vi "Example_OE2031&OE2041 Trig in_double_char.vi"() -> ()   [LabVIEW 2011]
panel:
  out "Wave":cluster{"Parameter":dbl, "Parameter":dbl}(graph)
  in  "Parameter Index2":u16(ring)=1 items=["X", "Y", "R", "θ", "Frequency", "XD1", "YD1", "RD1", "θD1", "XD2", "YD2", "RD2", "θD2", "XD3", "YD3", "RD3", "θD3", "X_Noise", "Y_Noise", "AUXADC1", "AUXADC2", "AUXADC3", "AUXADC4"]
  out "data_buffer":dbl[][](array[numeric])
  out "loss count":i32=-1
  out "cnt":u16
  in  "Ref_Source":u8(ring)=1 items=["External", "Internal"]
  in  "Interval Count":u32=1 min=1 max=100000
  in  "选项卡控件":enum32{"选项卡 "}(tab)
  in  "Sweep Mode":u16(ring) items=["Linear", "Log"]
  in  "Start Frequency(Hz)":dbl=1000.0 min=1e-05 max=60000000.0 format="%#.3f"
  in  "Stop Frequency(Hz)":dbl=5000.0 min=1e-05 max=60000000.0 format="%#.3f"
  in  "Linear Step Frequency(Hz)":dbl=1000.0 min=1e-05 max=60000000.0 format="%#.3f"
  in  "Log Step Percent(%)":dbl=10.0 min=-100.0 max=100.0 format="%#.2f"
  in  "Step Time(ms)":i32=1000 min=50 max=100000
  in  "Sweep Run Mode":u16(ring) items=["Stop", "Singal", "Loop"]
  out "Group":u32
  in  "Sweep":u16(ring) items=["OFF", "ON"]
  in  "function":T1(ring)
  in  "Parameter Index":u16(ring) items=["X", "Y", "R", "θ", "Frequency", "XD1", "YD1", "RD1", "θD1", "XD2", "YD2", "RD2", "θD2", "XD3", "YD3", "RD3", "θD3", "X_Noise", "Y_Noise", "AUXADC1", "AUXADC2", "AUXADC3", "AUXADC4"]
  in  "IP Address":string="192.168.1.10"
  in  "Timeout":u32=100
  in  "Port":u32=10001
  in  "Connect":bool
  in  "Trig Mode":u8(ring) items=["Internal", "Ext_Rissing_Edge", "Ext_Falling_Edge", "Ext_High_Level", "Ext_Low_Level"]
  out "Error out":errorcluster caption="error out"
  in  "Remote Mode":u16(ring) items=["USB"=0, "Ethernet"=3]
  in  "VISA resource name":refnum<visa-resource-name>
  # "Tel          :   +86-020-84133345\nWebsite  :   www.ssi-instrument.com\nE-mail     :   support@si-instrument.com"
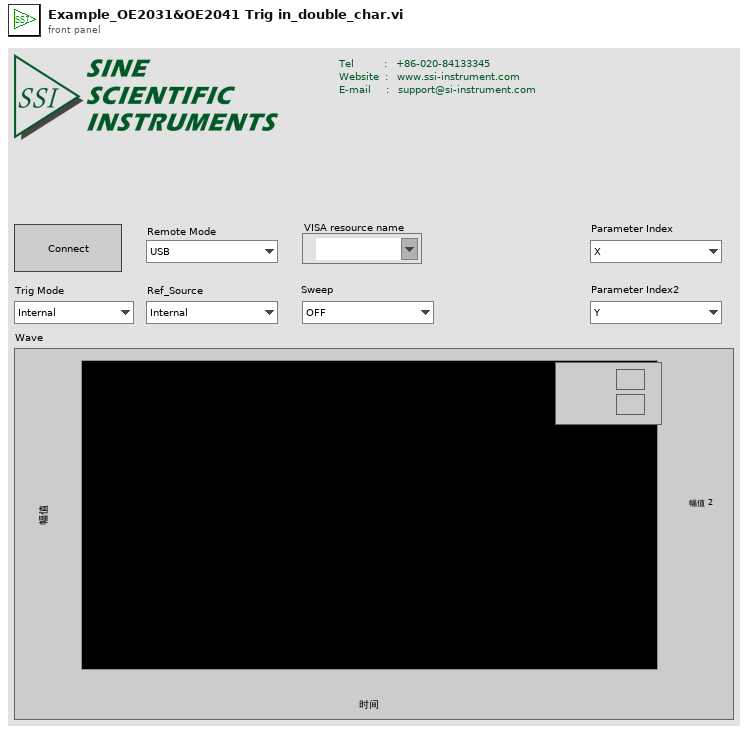
[diagram p1: front panel]
types:
  T1 = enum16{"initial", "Trig In Type", "Sample", "Ext_Sweep_Trig In", "Int_Sweep_Trig In"}
  T2 = enum8{"Enabled", "Disabled", "Disabled and Grayed Out"}
  T3 = cluster{"Port":u32, "Timeout":u32, "IP Address":string}
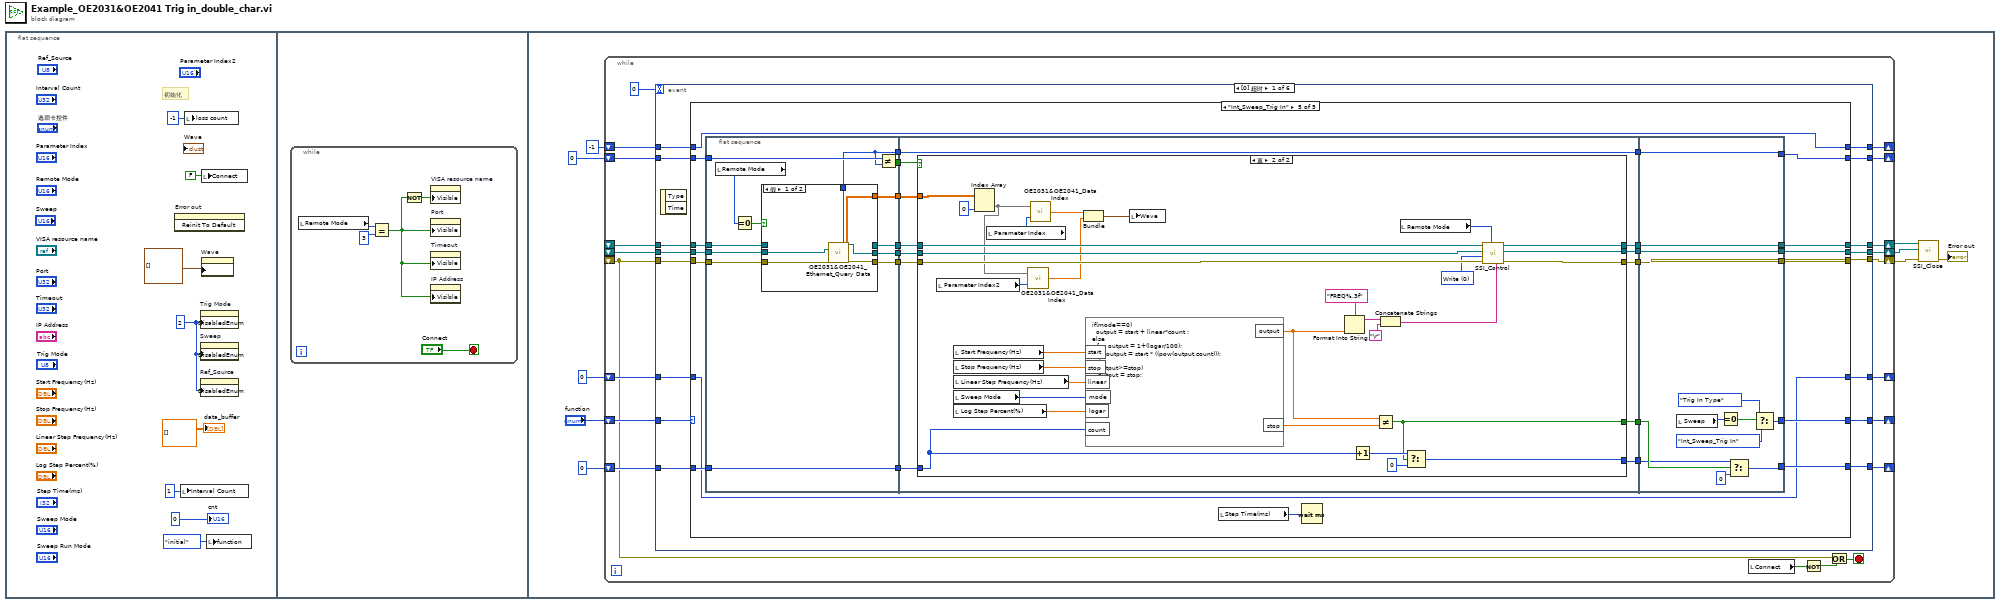
[diagram p0: block diagram]
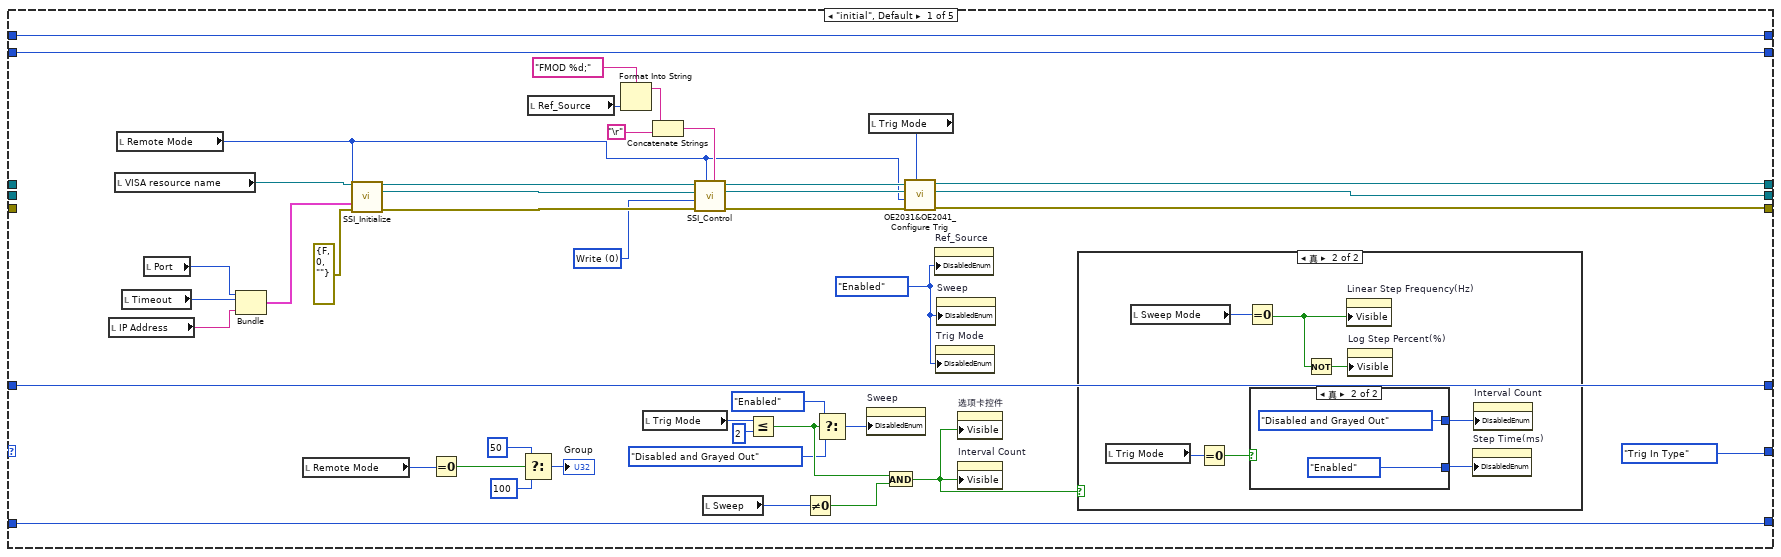
[diagram p2: hidden frame]
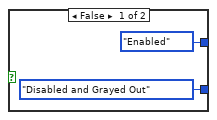
[diagram p4: hidden frame]
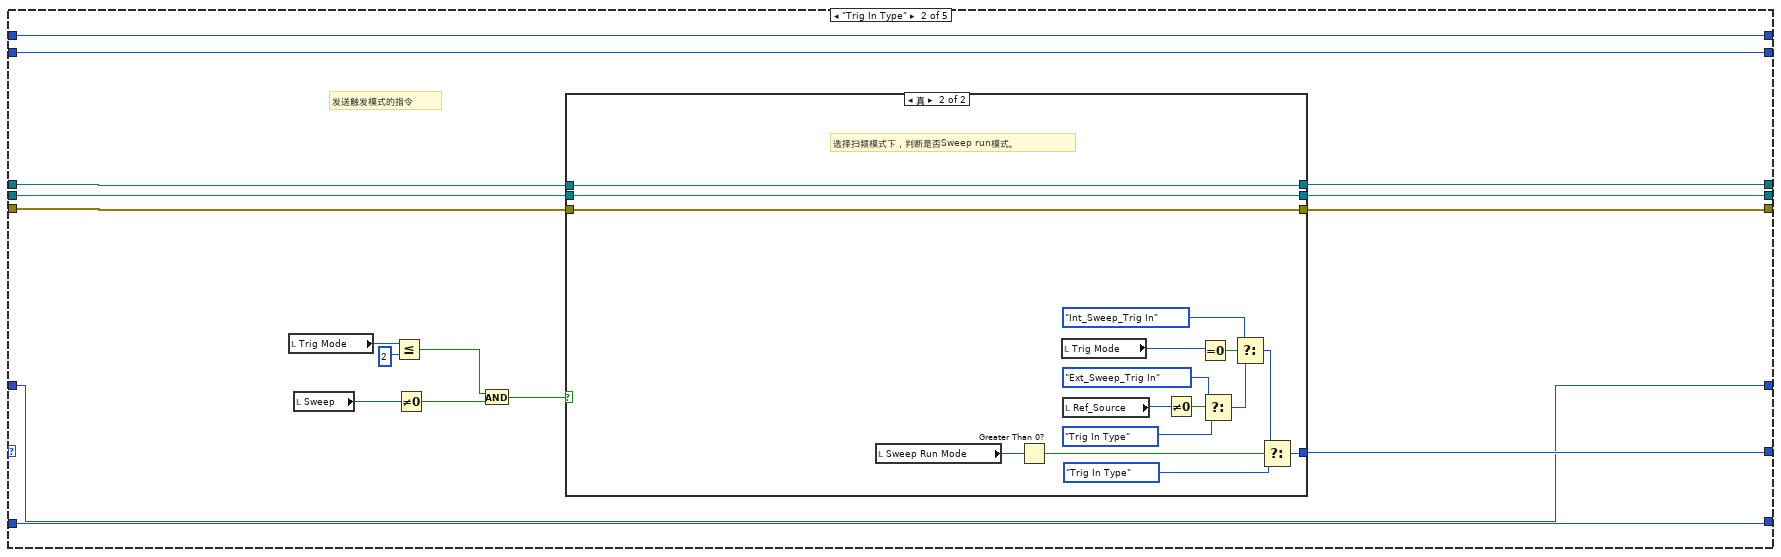
[diagram p5: hidden frame]
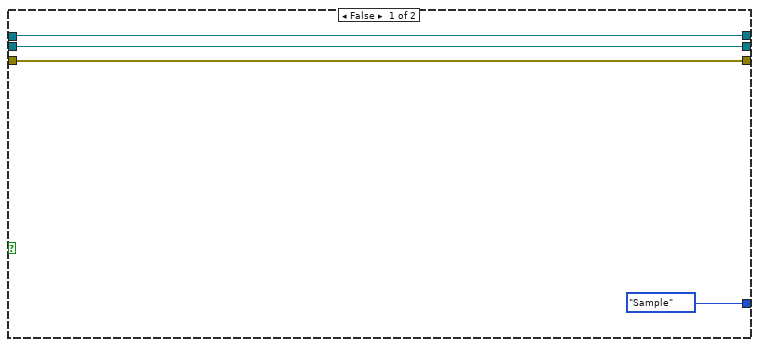
[diagram p6: hidden frame]
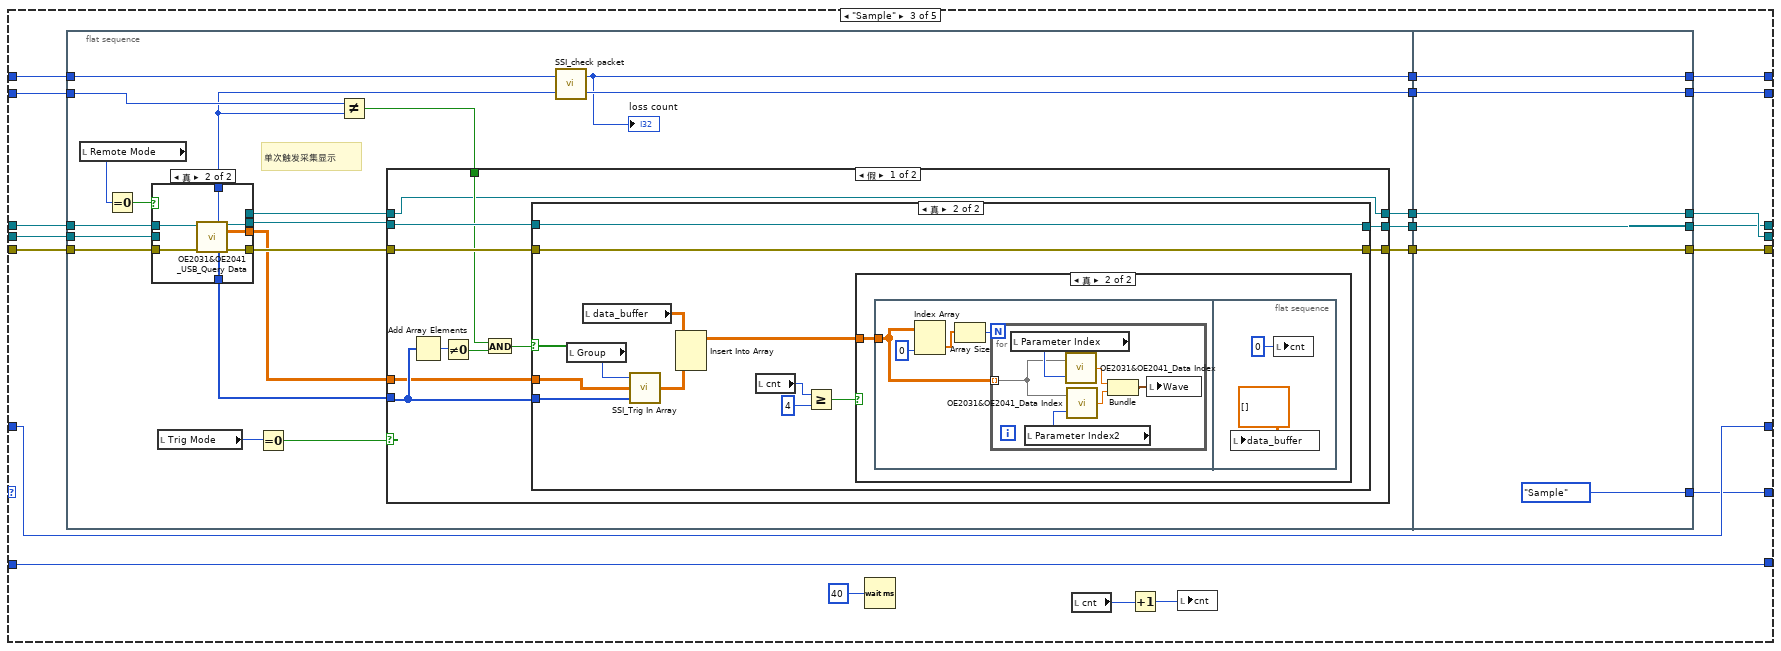
[diagram p7: hidden frame]
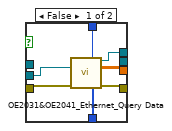
[diagram p8: hidden frame]
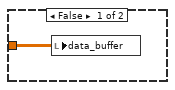
[diagram p10: hidden frame]
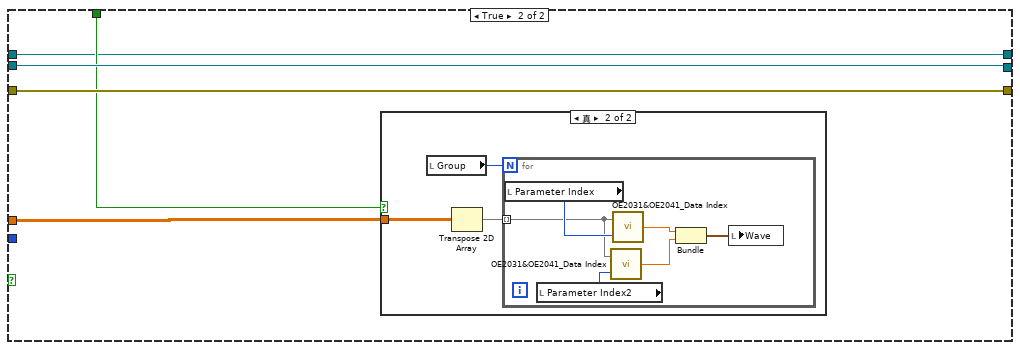
[diagram p11: hidden frame]
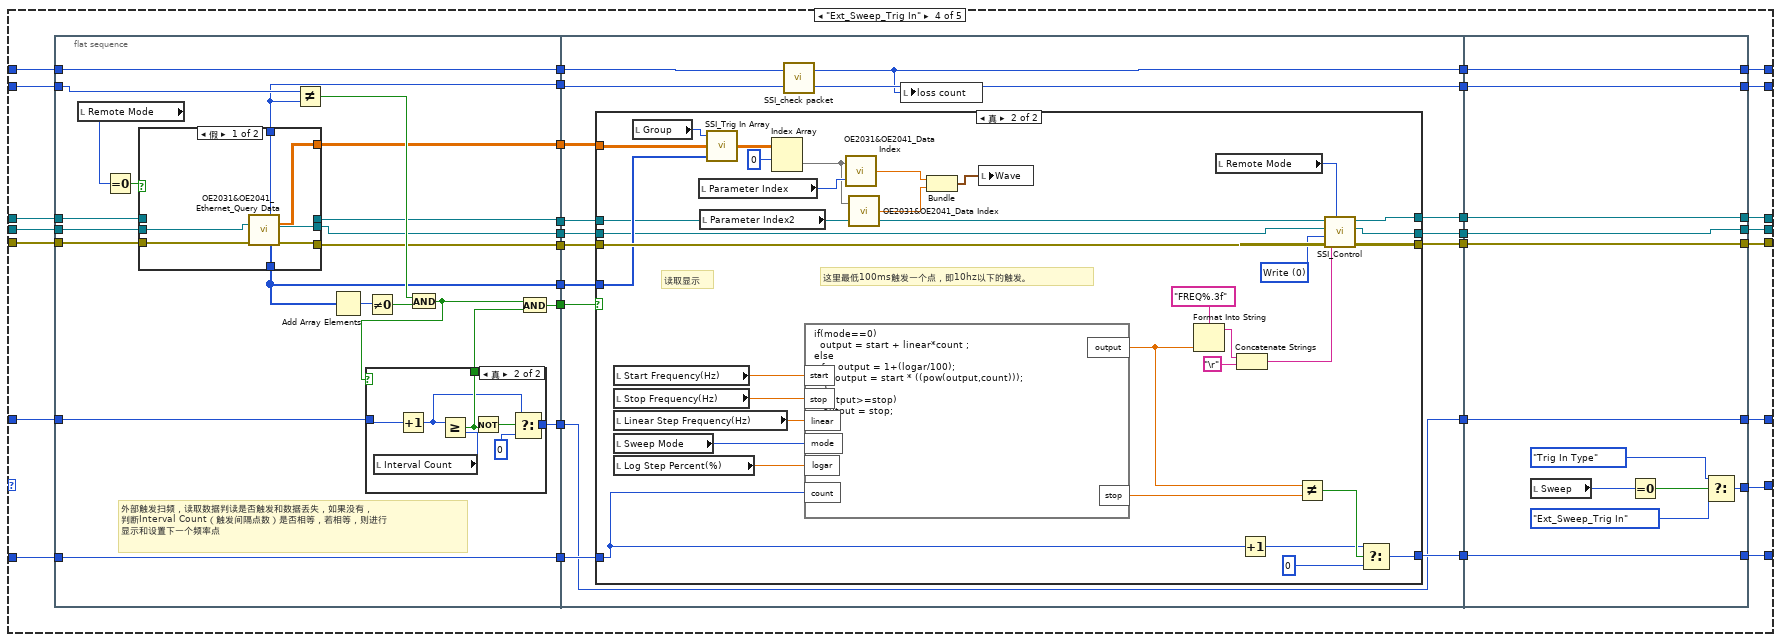
[diagram p13: hidden frame]
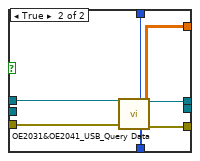
[diagram p14: hidden frame]
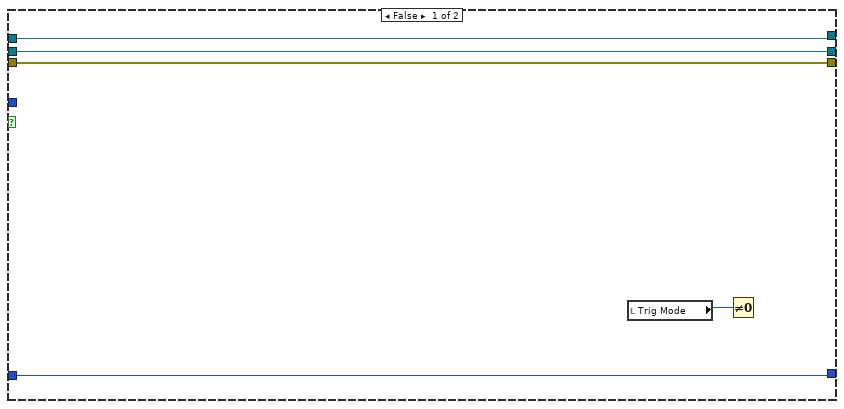
[diagram p16: hidden frame]
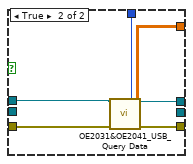
[diagram p17: hidden frame]
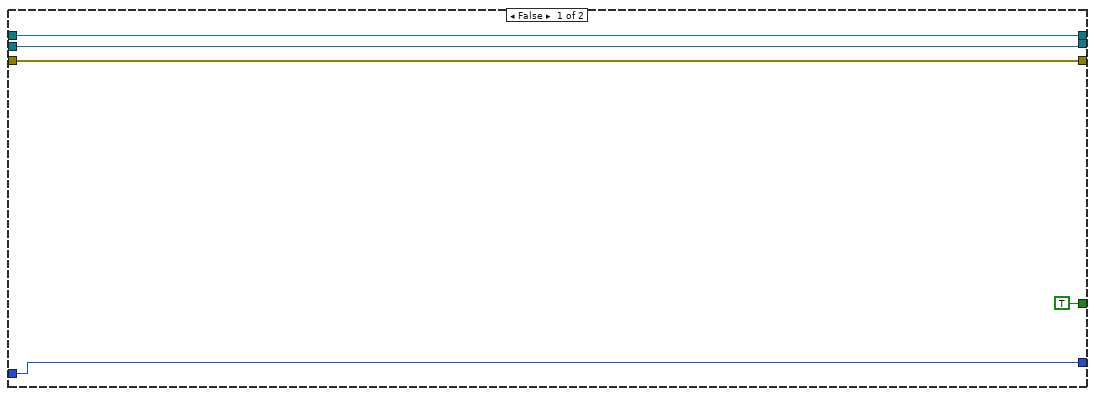
[diagram p18: hidden frame]
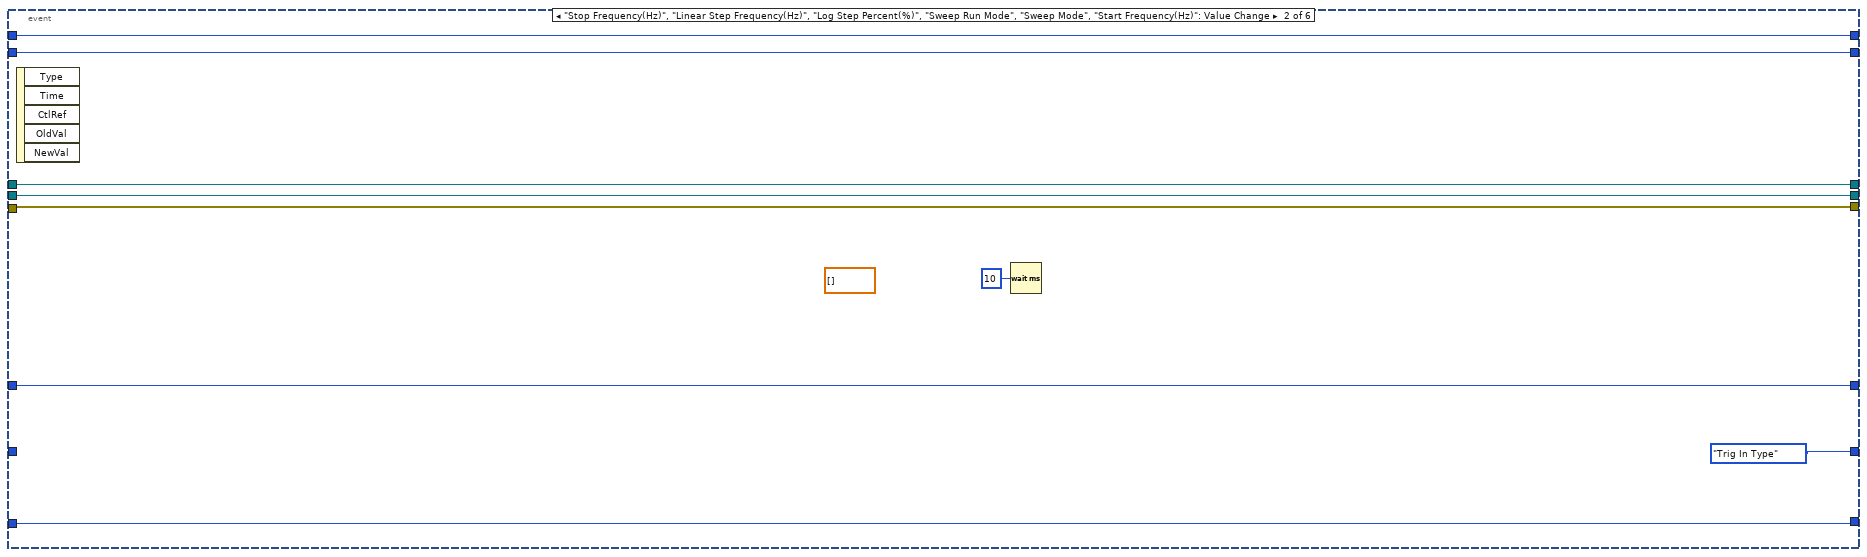
[diagram p19: hidden frame]
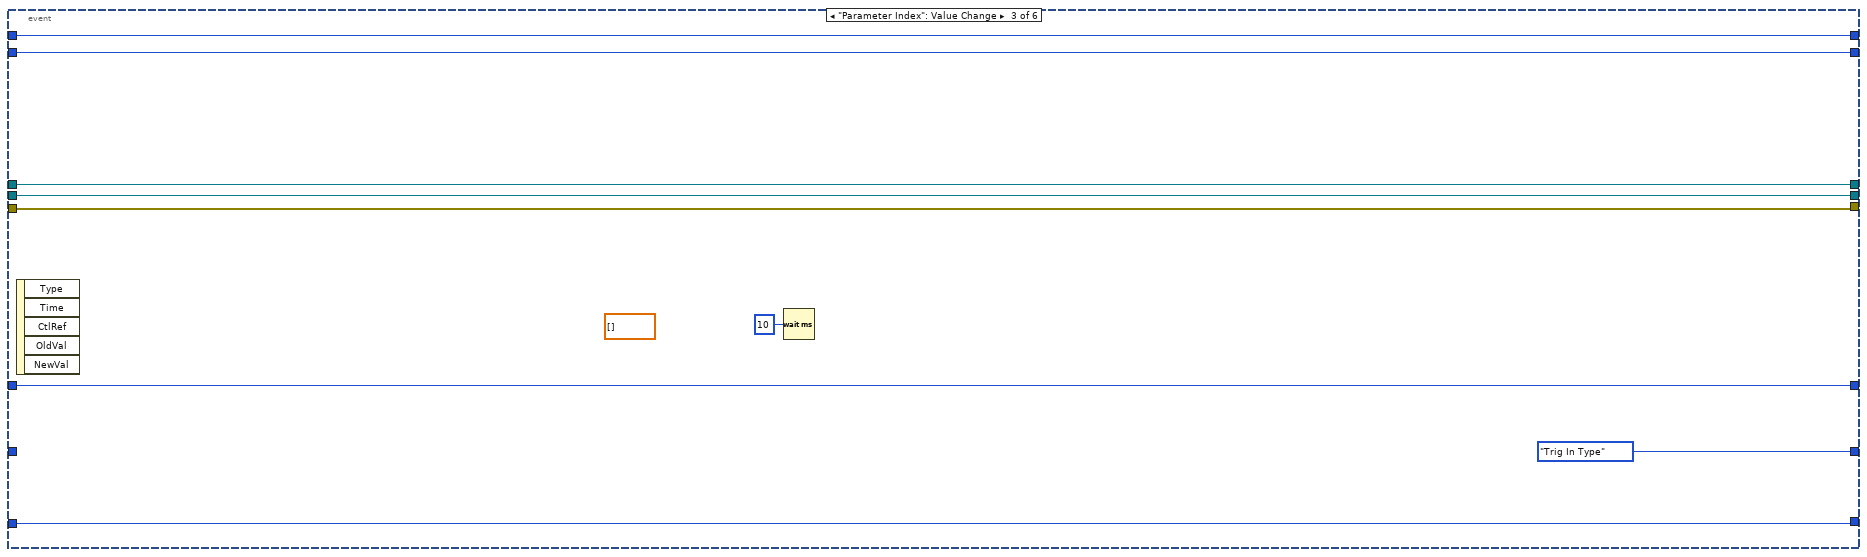
[diagram p20: hidden frame]
diagram:
  n1 = flat-sequence {
    frame #0 {
      w3 = 2
      # "初始化"
      n2 = invoke on="Error out" class="Clust (严格)" method="Reinit To Default"() -> ()  [unwired: 3 in, 3 out]
      n3 = local write "Interval Count"(u32 1 ("Interval Count")) -> ()
      n4 = local write "loss count"(-1 ("loss count")) -> ()
      n5 = property on="Trig Mode" class="Ring (严格)"("DisabledEnum"=w3) -> ()  [unwired: 2 in, 2 out]
      n6 = property on="Sweep" class="Ring (严格)"("DisabledEnum"=w3) -> ()  [unwired: 2 in, 2 out]
      n7 = property on="Ref_Source" class="Ring (严格)"("DisabledEnum"=w3) -> ()  [unwired: 2 in, 2 out]
      n8 = local write "Connect"(FALSE ("Connect")) -> ()
      n9 = property on="Wave" class="WFChart (严格)"("History Data"=cluster{"Parameter":dbl, "Parameter":dbl}[] [] ("历史数据")) -> ()  [unwired: 2 in, 2 out]
      n10 = local write "function"(T1."initial" ("function")) -> ()
      "data_buffer" <- dbl[][] []
      "cnt" <- 0
    }
    frame #1 {
      n11 = while {
        stop <- "Connect" stop-if-true
        n12 = local read "Remote Mode"() -> (w12:u16)
        n13 = Equal?(x=w12, y=u16 3) -> (x = y?=w10:bool)
        n14 = Not(x=w10) -> (.not. x?=w9:bool)
        n15 = property on="VISA resource name" class="VISAName"("Visible"=w9) -> ()  [unwired: 2 in, 2 out]
        n16 = property on="Port" class="DigNum (严格)"("Visible"=w10) -> ()  [unwired: 2 in, 2 out]
        n17 = property on="Timeout" class="DigNum (严格)"("Visible"=w10) -> ()  [unwired: 2 in, 2 out]
        n18 = property on="IP Address" class="Str"("Visible"=w10) -> ()  [unwired: 2 in, 2 out]
      }
    }
    frame #2 {
      n19 = while {
        shift-right: [w37] -> _
        shift-left: "function" -> [w38]
        shift-right: [w35] -> _
        shift-left: 0 ("f") -> [w36]
        shift-right: [w32] -> _
        shift-left: 0 -> [w33]
        shift-right: [w29] -> _
        shift-left: 0 -> [w30]
        shift-right: [w26] -> w16
        shift-left: _ -> [w40]
        shift-right: [w39] -> w21
        shift-left: _ -> [w28]
        shift-right: [w27] -> w17
        shift-left: _ -> [w25]
        shift-right: [w23] -> _
        shift-left: -1 ("loss count") -> [w24]
        stop <- w41 stop-if-true
        n20 = event shown="[0] 超时" {
          selector: _ -> [_ _ _ _ _ _]
          dyn-events: _ -> [_ _ _ _ _ _]
          timeout: 0 -> [_ _ _ _ _ _]
          tunnel: w40 -> [w58 w524 w536 w554 w578 w597]
          tunnel: [w57 w524 w536 w549 w577 w597] -> w26
          tunnel: [w56 w522 w535 w551 w580 w598] -> w39
          tunnel: w28 -> [w55 w522 w535 w556 w581 w598]
          tunnel: w38 -> [w54 _ _ _ w584 _]
          tunnel: [w53 T1."Trig In Type" ("function") T1."Trig In Type" ("function") T1."Trig In Type" ("function") w584 T1."Trig In Type" ("function")] -> w37
          tunnel: w36 -> [w52 w528 w537 w560 w585 w593]
          tunnel: [w51 w528 w537 w560 w585 w593] -> w35
          tunnel: w33 -> [w50 w526 w533 w558 w582 w595]
          tunnel: [w49 w526 w533 w558 w582 w595] -> w32
          tunnel: w30 -> [w48 w520 w532 w559 w583 w592]
          tunnel: [w47 w520 w532 w559 w583 w592] -> w29
          tunnel: [w46 w523 w530 w550 w576 w596] -> w27
          tunnel: w25 -> [w45 w523 w530 w555 w579 w596]
          tunnel: w24 -> [w44 w525 w529 w538 w572 w594]
          tunnel: [w43 w525 w529 w538 w572 w594] -> w23
          event Timeout {
            n21 = event-data() -> ()  [unwired: 1 in, 2 out]
            n22 = case shown="\"Int_Sweep_Trig In\"" w54 {
              tunnel: w58 -> [_ w129 w169 w294 w417]
              tunnel: w55 -> [_ w127 w168 w293 w416]
              tunnel: [w80 w128 w152 w290 w430] -> w57
              tunnel: [w78 w126 w160 w291 w429] -> w56
              tunnel: [T1."Trig In Type" ("function") w125 w166 w279 w427] -> w53
              tunnel: w52 -> [w95 w124 w170 w292 w428]
              tunnel: [w95 w124 w170 w289 w426] -> w51
              tunnel: w50 -> [w93 w123 w165 w288 w432]
              tunnel: [w93 w123 w163 w287 w431] -> w49
              tunnel: w48 -> [w94 w122 w167 w274 w425]
              tunnel: [w94 w122 w167 w271 w425] -> w47
              tunnel: [w79 w114 w153 w267 w408] -> w46
              tunnel: w45 -> [_ w115 w155 w270 w412]
              tunnel: w44 -> [w60 w113 w158 w266 w407]
              tunnel: [w60 w113 w151 w263 w407] -> w43
              frame "initial", Default {
                w59 = T2."Enabled" ("禁用")
                w72 = u16 0 items=["Write", "Read"] ("Control")
                n23 = local read "IP Address"() -> (w75:string)
                n24 = local read "VISA resource name"() -> (w81:refnum<visa-resource-name>)
                n25 = local read "Remote Mode"() -> (w61:u16)
                n26 = local read "Timeout"() -> (w76:u32)
                n27 = local read "Port"() -> (w77:u32)
                n28 = Bundle("Port"=w77, "Timeout"=w76, "IP Address"=w75) -> (w74:T3)  [unwired: 1 in]
                n29 = local read "Remote Mode"() -> (w101:u16)
                n30 = call "SSI_Initialize.vi"("VISA resource name"=w81, "Remote Mode"=w61, "Ethernet"=w74, "error in (no error)"=errorcluster {"status"=FALSE, "code"=0, "source"=""}) -> ("VISA resource name out"=w85:refnum<visa-resource-name>, "connection ID(Ethernet)"=w86:refnum<k5>, "error out"=w82:errorcluster)  [unwired: 9 in]
                n31 = Equal To 0?(x=w101) -> (x = 0?=w97:bool)
                n32 = Select(t=50, s=w97, f=100) -> (s? t:f=→"Group":i32)
                n33 = local read "Ref_Source"() -> (w91:u8)
                n34 = Format Into String(format string="FMOD %d;" ("格式字符串"), w91) -> (resulting string=w92:string)  [unwired: 2 in, 1 out]
                n35 = local read "Trig Mode"() -> (w67:u8)
                n36 = Concatenate Strings(w92, "\r") -> (w71:string)
                n37 = call "SSI_Control.vi"("Write Buffer"=w71, "Remote Mode"=w61, "Error in (no error)"=w82, "Control"=w72, "Connection ID in"=w86, "VISA resource name"=w85) -> ("Error out"=w83:errorcluster, "Connection ID out"=w84:refnum<k5>, "VISA resource  out"=w87:refnum<visa-resource-name>)  [unwired: 2 in, 1 out]
                n38 = local read "Sweep"() -> (w68:u16)
                n39 = Less Or Equal?(x=w67, y=u8 2) -> (x <= y?=w69:bool)
                n40 = Not Equal To 0?(x=w68) -> (x != 0?=w70:bool)
                n41 = Select(t=T2."Enabled" ("禁用"), s=w69, f=T2."Disabled and Grayed Out") -> (s? t:f=w64:T2)
                n42 = property on="Sweep" class="Ring (严格)"("DisabledEnum"=w64) -> ()  [unwired: 2 in, 2 out]
                n43 = local read "Trig Mode"() -> (w88:u8)
                n44 = And(x=w69, y=w70) -> (x .and. y?=w62:bool)
                n45 = call "OE2031&OE2041_Configure Trig.vi"("Trig Mode"=w88, "Error in (no error)"=w83, "Remote Mode"=w61, "Connection ID in"=w84, "VISA resource name"=w87) -> ("Error out"=w78:errorcluster, "Connection ID out"=w79:refnum<k5>, "VISA resource  out"=w80:refnum<visa-resource-name>)  [unwired: 3 in, 1 out]
                n46 = property on="Ref_Source" class="Ring (严格)"("DisabledEnum"=w59) -> ()  [unwired: 2 in, 2 out]
                n47 = property on="Trig Mode" class="Ring (严格)"("DisabledEnum"=w59) -> ()  [unwired: 2 in, 2 out]
                n48 = property on="Sweep" class="Ring (严格)"("DisabledEnum"=w59) -> ()  [unwired: 2 in, 2 out]
                n49 = property on="选项卡控件" class="TabCtl (严格)"("Visible"=w62) -> ()  [unwired: 2 in, 2 out]
                n50 = property on="Interval Count" class="DigNum (严格)"("Visible"=w62) -> ()  [unwired: 2 in, 2 out]
                n51 = case shown="真" w62 {
                  frame False {
                  }
                  frame True {
                    n52 = local read "Trig Mode"() -> (w102:u8)
                    n53 = local read "Sweep Mode"() -> (w107:u16)
                    n54 = Equal To 0?(x=w102) -> (x = 0?=w103:bool)
                    n55 = Equal To 0?(x=w107) -> (x = 0?=w108:bool)
                    n56 = case shown="真" w103 {
                      tunnel: [T2."Disabled and Grayed Out" ("禁用") T2."Enabled" ("禁用")] -> w105
                      tunnel: [T2."Enabled" ("禁用") T2."Disabled and Grayed Out" ("禁用")] -> w104
                      frame False {
                      }
                      frame True {
                      }
                    }
                    n57 = Not(x=w108) -> (.not. x?=w106:bool)
                    n58 = property on="Linear Step Frequency(Hz)" class="DigNum (严格)"("Visible"=w108) -> ()  [unwired: 2 in, 2 out]
                    n59 = property on="Log Step Percent(%)" class="DigNum (严格)"("Visible"=w106) -> ()  [unwired: 2 in, 2 out]
                    n60 = property on="Step Time(ms)" class="DigNum (严格)"("DisabledEnum"=w105) -> ()  [unwired: 2 in, 2 out]
                    n61 = property on="Interval Count" class="DigNum (严格)"("DisabledEnum"=w104) -> ()  [unwired: 2 in, 2 out]
                  }
                }
              }
              frame "Trig In Type" {
                # "发送触发模式的指令"
                n62 = local read "Trig Mode"() -> (w119:u8)
                n63 = local read "Sweep"() -> (w118:u16)
                n64 = Less Or Equal?(x=w119, y=u8 2) -> (x <= y?=w117:bool)
                n65 = Not Equal To 0?(x=w118) -> (x != 0?=w116:bool)
                n66 = And(x=w117, y=w116) -> (x .and. y?=w121:bool)
                n67 = case shown="真" w121 {
                  tunnel: [w133 w145] -> w128
                  tunnel: [w132 w144] -> w126
                  tunnel: w127 -> [w132 w144]
                  tunnel: w129 -> [w133 w145]
                  tunnel: [T1."Sample" ("function") w148] -> w125
                  tunnel: w115 -> [w130 w134]
                  tunnel: [w130 w134] -> w114
                  frame False {
                  }
                  frame True {
                    # "选择扫频模式下，判断是否Sweep run模式。"
                    n68 = local read "Sweep Run Mode"() -> (w146:u16)
                    n69 = Greater Than 0?(x=w146) -> (x > 0?=w149:bool)
                    n70 = local read "Trig Mode"() -> (w139:u8)
                    n71 = local read "Ref_Source"() -> (w143:u8)
                    n72 = Not Equal To 0?(x=w143) -> (x != 0?=w142:bool)
                    n73 = Equal To 0?(x=w139) -> (x = 0?=w140:bool)
                    n74 = Select(t=T1."Ext_Sweep_Trig In" ("function"), s=w142, f=T1."Trig In Type" ("function")) -> (s? t:f=w141:T1)
                    n75 = Select(t=T1."Int_Sweep_Trig In" ("function"), s=w140, f=w141) -> (s? t:f=w147:T1)
                    n76 = Select(t=w147, s=w149, f=T1."Trig In Type" ("function")) -> (s? t:f=w148:T1)
                  }
                }
              }
              frame "Sample" {
                n77 = flat-sequence {
                  tunnel: w169 -> [w189]
                  tunnel: w168 -> [w188]
                  tunnel: w165 -> [w185]
                  tunnel: [w181] -> w164
                  tunnel: [w183] -> w162
                  tunnel: [w182] -> w161
                  tunnel: w158 -> [w180]
                  tunnel: w155 -> [w176]
                  tunnel: [w173] -> w154
                  tunnel: [w172] -> w150
                  tunnel: w164 -> [w258]
                  tunnel: w162 -> [w262]
                  tunnel: w161 -> [w261]
                  tunnel: [T1."Sample" ("function")] -> w166
                  tunnel: [w258] -> w163
                  tunnel: [w262] -> w152
                  tunnel: [w261] -> w160
                  tunnel: w154 -> [w259]
                  tunnel: [w259] -> w153
                  tunnel: [w257] -> w151
                  tunnel: w150 -> [w257]
                  frame #0 {
                    # "单次触发采集显示"
                    n78 = local read "Remote Mode"() -> (w177:u16)
                    n79 = Equal To 0?(x=w177) -> (x = 0?=w178:bool)
                    n80 = case shown="真" w178 {
                      tunnel: w189 -> [_ w204]
                      tunnel: w188 -> [w196 w203]
                      tunnel: [w193 w202] -> w186
                      tunnel: [w197 w201] -> w184
                      tunnel: [w192 w200] -> w181
                      tunnel: [w194 w199] -> w179
                      tunnel: w176 -> [w195 _]
                      tunnel: [_ w198] -> w175
                      tunnel: [w191 _] -> w174
                      frame False {
                        n81 = call "OE2031&OE2041_Ethernet_Query Data.vi"("Connection ID in"=w195, "Error in (no error)"=w196) -> ("Buffer Count"=w192:u8, "Connection ID out"=w191:refnum<k5>, "Total Data Array"=w194:dbl[][], "Trig In_Count"=w193:u8[], "Error out"=w197:errorcluster)  [unwired: 6 in, 3 out]
                      }
                      frame True {
                        n82 = call "OE2031&OE2041_USB_Query Data.vi"("VISA resource name"=w204, "Error in (no error)"=w203) -> ("Buffer Count"=w200:u8, "VISA resource  out"=w198:refnum<visa-resource-name>, "Total Data Array"=w199:dbl[][], "Trig In_Count"=w202:u8[], "Error out"=w201:errorcluster)  [unwired: 6 in, 3 out]
                      }
                    }
                    n83 = local read "Trig Mode"() -> (w190:u8)
                    n84 = Equal To 0?(x=w190) -> (x = 0?=w187:bool)
                    n85 = Not Equal?(x=w185, y=w181) -> (x != y?=w171:bool)
                    n86 = case shown="假" w187 {
                      tunnel: w179 -> [w207 w245]
                      tunnel: w186 -> [w214 _]
                      tunnel: w171 -> [w206 w244]
                      tunnel: w184 -> [w209 w246]
                      tunnel: w175 -> [w211 w247]
                      tunnel: [w210 w247] -> w183
                      tunnel: [w208 w246] -> w182
                      tunnel: w174 -> [w205 w243]
                      tunnel: [w205 w243] -> w173
                      frame False {
                        n87 = Add Array Elements(numeric array=w214) -> (sum=w215:u8)
                        n88 = Not Equal To 0?(x=w215) -> (x != 0?=w213:bool)
                        n89 = And(x=w206, y=w213) -> (x .and. y?=w212:bool)
                        n90 = case shown="真" w212 {
                          tunnel: w207 -> [_ w226]
                          tunnel: w214 -> [_ w225]
                          tunnel: [w217 w228] -> w210
                          tunnel: w211 -> [w217 w228]
                          tunnel: w209 -> [w216 w227]
                          tunnel: [w216 w227] -> w208
                          frame False {
                          }
                          frame True {
                            n91 = local read "Group"() -> (w224:u32)
                            n92 = local read "data_buffer"() -> (w223:dbl[][])
                            n93 = call "SSI_Trig In Array.vi"("Trig_Count"=w225, "Input Array"=w226, "Group"=w224) -> ("Output Array"=w222:dbl[][])
                            n94 = Insert Into Array(array=w223, new element=w222) -> (w221:dbl[][])  [unwired: 2 in]
                            n95 = local read "cnt"() -> (w220:u16)
                            n96 = Greater Or Equal?(x=w220, y=u16 4) -> (x >= y?=w218:bool)
                            n97 = case shown="真" w218 {
                              tunnel: w221 -> [w229 w230]
                              frame False {
                                n98 = local write "data_buffer"(w229) -> ()
                              }
                              frame True {
                                n99 = flat-sequence {
                                tunnel: w230 -> [w232]
                                frame #0 {
                                n100 = Index Array(array=w232, index (col)=0 ("禁用的索引 (列)")) -> (element=w231:dbl[])  [unwired: 1 in]
                                n101 = Array Size(array=w231) -> (size(s)=w234:i32)
                                n102 = for {
                                N: w234 -> [_]
                                tunnel: w232 -> [w239] mode=indexing
                                n103 = local read "Parameter Index"() -> (w240:u16)
                                n104 = local read "Parameter Index2"() -> (w235:u16)
                                n105 = call "OE2031&OE2041_Data Index.vi"("Parameter Type"=w240, "Input Date Array"=w239) -> ("Parameter"=w238:dbl)
                                n106 = call "OE2031&OE2041_Data Index.vi"("Parameter Type"=w235, "Input Date Array"=w239) -> ("Parameter"=w237:dbl)
                                n107 = Bundle("Parameter"=w238, "Parameter"=w237) -> (w236:cluster{"Parameter":dbl, "Parameter":dbl})  [unwired: 1 in]
                                n108 = local write "Wave"(w236) -> ()
                                }
                                }
                                frame #1 {
                                n109 = local write "data_buffer"(dbl[][] [] ("data_buffer")) -> ()
                                n110 = local write "cnt"(u16 0 ("cnt")) -> ()
                                }
                                }
                              }
                            }
                          }
                        }
                      }
                      frame True {
                        n111 = case shown="真" w244 {
                          tunnel: w245 -> [_ w250]
                          frame False {
                          }
                          frame True {
                            n112 = local read "Group"() -> (w249:u32)
                            n113 = Transpose 2D Array(2D array=w250) -> (transposed array=w248:dbl[][])
                            n114 = for {
                              N: w249 -> [_]
                              tunnel: w248 -> [w255] mode=indexing
                              n115 = local read "Parameter Index"() -> (w256:u16)
                              n116 = local read "Parameter Index2"() -> (w254:u16)
                              n117 = call "OE2031&OE2041_Data Index.vi"("Parameter Type"=w254, "Input Date Array"=w255) -> ("Parameter"=w252:dbl)
                              n118 = call "OE2031&OE2041_Data Index.vi"("Parameter Type"=w256, "Input Date Array"=w255) -> ("Parameter"=w253:dbl)
                              n119 = Bundle("Parameter"=w253, "Parameter"=w252) -> (w251:cluster{"Parameter":dbl, "Parameter":dbl})  [unwired: 1 in]
                              n120 = local write "Wave"(w251) -> ()
                            }
                          }
                        }
                      }
                    }
                    n121 = call "SSI_check packet.vi"("input"=w181, "input loss"=w180) -> ("loss count"=w172:i32)  [unwired: 1 out]
                    "loss count" <- w172
                  }
                  frame #1 {
                  }
                }
                n122 = Wait (ms)(milliseconds to wait=40) -> ()  [unwired: 1 out]
                n123 = local read "cnt"() -> (w156:u16)
                n124 = Increment(x=w156) -> (x+1=w157:u16)
                n125 = local write "cnt"(w157) -> ()
              }
              frame "Ext_Sweep_Trig In" {
                n126 = flat-sequence {
                  tunnel: w294 -> [w315]
                  tunnel: w293 -> [w314]
                  tunnel: w292 -> [w312]
                  tunnel: [w308] -> w286
                  tunnel: w288 -> [w316]
                  tunnel: [w312] -> w285
                  tunnel: [w313] -> w284
                  tunnel: [w307] -> w278
                  tunnel: [w306] -> w277
                  tunnel: [w305] -> w276
                  tunnel: [w304] -> w275
                  tunnel: w274 -> [w302]
                  tunnel: [w300] -> w273
                  tunnel: w270 -> [w297]
                  tunnel: [w296] -> w269
                  tunnel: w266 -> [w295]
                  tunnel: [w295] -> w265
                  tunnel: w286 -> [w353]
                  tunnel: w284 -> [w340]
                  tunnel: w285 -> [w349]
                  tunnel: [w350] -> w283
                  tunnel: [w351] -> w282
                  tunnel: [w348] -> w281
                  tunnel: [w340] -> w280
                  tunnel: w278 -> [w352]
                  tunnel: w277 -> [w347]
                  tunnel: w276 -> [w346]
                  tunnel: w275 -> [w345]
                  tunnel: w273 -> [w344]
                  tunnel: [w344] -> w272
                  tunnel: w269 -> [w343]
                  tunnel: [w342] -> w268
                  tunnel: w265 -> [w341]
                  tunnel: [w339] -> w264
                  tunnel: [w404] -> w287
                  tunnel: [w405] -> w289
                  tunnel: [w402] -> w290
                  tunnel: [w403] -> w291
                  tunnel: w283 -> [w403]
                  tunnel: w282 -> [w402]
                  tunnel: w281 -> [w405]
                  tunnel: w280 -> [w404]
                  tunnel: [w400] -> w279
                  tunnel: w272 -> [w401]
                  tunnel: [w401] -> w271
                  tunnel: w268 -> [w395]
                  tunnel: [w395] -> w267
                  tunnel: w264 -> [w394]
                  tunnel: [w394] -> w263
                  frame #0 {
                    # "外部触发扫频，读取数据判读是否触发和数据丢失，如果没有，\n判断Interval Count（触发间隔点数）是否相等，若相等，则进行\n显示和设置下一个频率点"
                    n127 = local read "Remote Mode"() -> (w298:u16)
                    n128 = Equal To 0?(x=w298) -> (x = 0?=w299:bool)
                    n129 = case shown="假" w299 {
                      tunnel: w315 -> [_ w330]
                      tunnel: w314 -> [w323 w329]
                      tunnel: [w319 w328] -> w313
                      tunnel: [_ w327] -> w308
                      tunnel: [w322 w326] -> w307
                      tunnel: [w320 w325] -> w306
                      tunnel: [w318 w324] -> w305
                      tunnel: [w321 _] -> w296
                      tunnel: w297 -> [w317 _]
                      frame False {
                        n130 = call "OE2031&OE2041_Ethernet_Query Data.vi"("Connection ID in"=w317, "Error in (no error)"=w323) -> ("Buffer Count"=w319:u8, "Connection ID out"=w321:refnum<k5>, "Total Data Array"=w320:dbl[][], "Trig In_Count"=w318:u8[], "Error out"=w322:errorcluster)  [unwired: 6 in, 3 out]
                      }
                      frame True {
                        n131 = call "OE2031&OE2041_USB_Query Data.vi"("VISA resource name"=w330, "Error in (no error)"=w329) -> ("Buffer Count"=w328:u8, "VISA resource  out"=w327:refnum<visa-resource-name>, "Total Data Array"=w325:dbl[][], "Trig In_Count"=w324:u8[], "Error out"=w326:errorcluster)  [unwired: 6 in, 3 out]
                      }
                    }
                    n132 = Not Equal?(x=w316, y=w313) -> (x != y?=w310:bool)
                    n133 = Add Array Elements(numeric array=w305) -> (sum=w311:u8)
                    n134 = Not Equal To 0?(x=w311) -> (x != 0?=w309:bool)
                    n135 = And(x=w310, y=w309) -> (x .and. y?=w303:bool)
                    n136 = case shown="真" w303 {
                      tunnel: w302 -> [w331 w338]
                      tunnel: [_ w335] -> w301
                      tunnel: [w331 w332] -> w300
                      frame False {
                      }
                      frame True {
                        n137 = local read "Interval Count"() -> (w337:u32)
                        n138 = Increment(x=w338) -> (x+1=w334:i32)
                        n139 = Greater Or Equal?(x=w334, y=w337) -> (x >= y?=w335:bool)
                        n140 = Not(x=w335) -> (.not. x?=w336:bool)
                        n141 = Select(t=w334, s=w336, f=0) -> (s? t:f=w332:i32)
                      }
                    }
                    n142 = And(x=w303, y=w301) -> (x .and. y?=w304:bool)
                  }
                  frame #1 {
                    n143 = case shown="真" w345 {
                      tunnel: w352 -> [w357 w376]
                      tunnel: [w357 w378] -> w350
                      tunnel: [w358 w365] -> w351
                      tunnel: w353 -> [w358 w366]
                      tunnel: w349 -> [w356 w384]
                      tunnel: [w356 w383] -> w348
                      tunnel: w347 -> [_ w374]
                      tunnel: w346 -> [_ w372]
                      tunnel: w343 -> [w354 w370]
                      tunnel: [w354 w369] -> w342
                      frame False {
                        n144 = local read "Trig Mode"() -> (w355:u8)
                        n145 = Not Equal To 0?(x=w355) -> ()  [unwired: 1 out]
                      }
                      frame True {
                        w367 = u16 0 items=["Write", "Read"] ("Control")
                        # "这里最低100ms触发一个点，即10hz以下的触发。"
                        # "读取显示"
                        n146 = local read "Start Frequency(Hz)"() -> (w390:dbl)
                        n147 = local read "Stop Frequency(Hz)"() -> (w389:dbl)
                        n148 = local read "Linear Step Frequency(Hz)"() -> (w388:dbl)
                        n149 = local read "Sweep Mode"() -> (w387:u16)
                        n150 = local read "Log Step Percent(%)"() -> (w386:dbl)
                        n151 = local read "Group"() -> (w373:u32)
                        n152 = local read "Parameter Index"() -> (w375:u16)
                        n153 = local read "Parameter Index2"() -> (w362:u16)
                        n154 = call "SSI_Trig In Array.vi"("Trig_Count"=w372, "Input Array"=w374, "Group"=w373) -> ("Output Array"=w371:dbl[][])
                        n155 = Index Array(array=w371, index (row)=0 ("索引 (行)")) -> (element=w363:dbl[])  [unwired: 1 in]
                        n156 = formula code="if(mode==0)\n  output = start + linear*count ;\nelse \n  {    output = 1+(logar/100);\n       output = start * ((pow(output,count)));\n   }\nif(output>=stop)\n   output = stop;"("start"=w390, "stop"=w389, "linear"=w388, "logar"=w386, "mode"=w387, "count"=w384) -> ("stop"=w385:dbl, "output"=w379:dbl)
                        n157 = call "OE2031&OE2041_Data Index.vi"("Parameter Type"=w375, "Input Date Array"=w363) -> ("Parameter"=w361:dbl)
                        n158 = call "OE2031&OE2041_Data Index.vi"("Parameter Type"=w362, "Input Date Array"=w363) -> ("Parameter"=w360:dbl)
                        n159 = Bundle("Parameter"=w361, "Parameter"=w360) -> (w359:cluster{"Parameter":dbl, "Parameter":dbl})  [unwired: 1 in]
                        n160 = local write "Wave"(w359) -> ()
                        n161 = Format Into String(format string="FREQ%.3f" ("格式字符串"), w379) -> (resulting string=w392:string)  [unwired: 2 in, 1 out]
                        n162 = local read "Remote Mode"() -> (w368:u16)
                        n163 = Concatenate Strings(w392, "\r") -> (w377:string)
                        n164 = Increment(x=w384) -> (x+1=w381:i32)
                        n165 = Not Equal?(x=w379, y=w385) -> (x != y?=w382:bool)
                        n166 = call "SSI_Control.vi"("Write Buffer"=w377, "Remote Mode"=w368, "Error in (no error)"=w376, "Control"=w367, "Connection ID in"=w370, "VISA resource name"=w366) -> ("Error out"=w378:errorcluster, "Connection ID out"=w369:refnum<k5>, "VISA resource  out"=w365:refnum<visa-resource-name>)  [unwired: 2 in, 1 out]
                        n167 = Select(t=w381, s=w382, f=0) -> (s? t:f=w383:i32)
                      }
                    }
                    n168 = call "SSI_check packet.vi"("input"=w340, "input loss"=w341) -> ("loss count"=w339:i32)  [unwired: 1 out]
                    n169 = local write "loss count"(w339) -> ()
                  }
                  frame #2 {
                    n170 = local read "Sweep"() -> (w399:u16)
                    n171 = Equal To 0?(x=w399) -> (x = 0?=w398:bool)
                    n172 = Select(t=T1."Trig In Type" ("function"), s=w398, f=T1."Ext_Sweep_Trig In" ("function")) -> (s? t:f=w400:T1)
                  }
                }
              }
              frame "Int_Sweep_Trig In" {
                n173 = flat-sequence {
                  tunnel: [w442] -> w424
                  tunnel: [w437] -> w422
                  tunnel: [w441] -> w420
                  tunnel: w432 -> [w445]
                  tunnel: w428 -> [w443]
                  tunnel: w417 -> [w438]
                  tunnel: w416 -> [w440]
                  tunnel: [w444] -> w415
                  tunnel: [w443] -> w414
                  tunnel: w412 -> [w439]
                  tunnel: [w436] -> w411
                  tunnel: [w433] -> w410
                  tunnel: w424 -> [w469]
                  tunnel: [w469] -> w423
                  tunnel: w422 -> [w468]
                  tunnel: [w467] -> w421
                  tunnel: w420 -> [w466]
                  tunnel: [w465] -> w419
                  tunnel: [w461] -> w418
                  tunnel: w415 -> [w464]
                  tunnel: w414 -> [w463]
                  tunnel: [w462] -> w413
                  tunnel: w411 -> [w460]
                  tunnel: w410 -> [w459]
                  tunnel: [w458] -> w409
                  tunnel: [w519] -> w431
                  tunnel: w423 -> [w519]
                  tunnel: w421 -> [w518]
                  tunnel: [w518] -> w430
                  tunnel: [w517] -> w429
                  tunnel: w419 -> [w517]
                  tunnel: [w510] -> w427
                  tunnel: [w516] -> w426
                  tunnel: w418 -> [w514]
                  tunnel: w413 -> [w513]
                  tunnel: w409 -> [w507]
                  tunnel: [w507] -> w408
                  frame #0 {
                    n174 = local read "Remote Mode"() -> (w434:u16)
                    n175 = Equal To 0?(x=w434) -> (x = 0?=w435:bool)
                    n176 = case shown="假" w435 {
                      tunnel: [w449 w457] -> w442
                      tunnel: [_ w456] -> w437
                      tunnel: [w451 w455] -> w441
                      tunnel: [w450 w454] -> w436
                      tunnel: w440 -> [w448 w452]
                      tunnel: w439 -> [w447 _]
                      tunnel: w438 -> [_ w453]
                      tunnel: [w446 _] -> w433
                      frame False {
                        n177 = call "OE2031&OE2041_Ethernet_Query Data.vi"("Connection ID in"=w447, "Error in (no error)"=w448) -> ("Buffer Count"=w449:u8, "Connection ID out"=w446:refnum<k5>, "Total Data Array"=w450:dbl[][], "Error out"=w451:errorcluster)  [unwired: 6 in, 4 out]
                      }
                      frame True {
                        n178 = call "OE2031&OE2041_USB_Query Data.vi"("VISA resource name"=w453, "Error in (no error)"=w452) -> ("Buffer Count"=w457:u8, "VISA resource  out"=w456:refnum<visa-resource-name>, "Total Data Array"=w454:dbl[][], "Error out"=w455:errorcluster)  [unwired: 6 in, 4 out]
                      }
                    }
                    n179 = Not Equal?(x=w445, y=w442) -> (x != y?=w444:bool)
                  }
                  frame #1 {
                    n180 = case shown="真" w464 {
                      tunnel: w468 -> [w474 w482]
                      tunnel: [w474 w481] -> w467
                      tunnel: [w473 w488] -> w465
                      tunnel: w466 -> [w473 w489]
                      tunnel: w463 -> [w472 w500]
                      tunnel: [w472 w494] -> w462
                      tunnel: [TRUE w495] -> w461
                      tunnel: w460 -> [_ w485]
                      tunnel: w459 -> [w470 w484]
                      tunnel: [w470 w480] -> w458
                      frame False {
                      }
                      frame True {
                        w483 = u16 0 items=["Write", "Read"] ("Control")
                        n181 = local read "Parameter Index2"() -> (w478:u16)
                        n182 = local read "Start Frequency(Hz)"() -> (w506:dbl)
                        n183 = local read "Stop Frequency(Hz)"() -> (w505:dbl)
                        n184 = local read "Linear Step Frequency(Hz)"() -> (w504:dbl)
                        n185 = local read "Sweep Mode"() -> (w503:u16)
                        n186 = local read "Log Step Percent(%)"() -> (w502:dbl)
                        n187 = Index Array(array=w485, index (col)=0 ("禁用的索引 (列)")) -> (element=w479:dbl[])  [unwired: 1 in]
                        n188 = local read "Parameter Index"() -> (w491:u16)
                        n189 = call "OE2031&OE2041_Data Index.vi"("Parameter Type"=w478, "Input Date Array"=w479) -> ("Parameter"=w476:dbl)
                        n190 = call "OE2031&OE2041_Data Index.vi"("Parameter Type"=w491, "Input Date Array"=w479) -> ("Parameter"=w477:dbl)
                        n191 = Bundle("Parameter"=w477, "Parameter"=w476) -> (w475:cluster{"Parameter":dbl, "Parameter":dbl})  [unwired: 1 in]
                        n192 = formula code="if(mode==0)\n  output = start + linear*count ;\nelse \n  {    output = 1+(logar/100);\n       output = start * ((pow(output,count)));\n   }\nif(output>=stop)\n   output = stop;"("start"=w506, "stop"=w505, "linear"=w504, "logar"=w502, "mode"=w503, "count"=w500) -> ("stop"=w496:dbl, "output"=w492:dbl)
                        n193 = local write "Wave"(w475) -> ()
                        n194 = Format Into String(format string="FREQ%.3f" ("格式字符串"), w492) -> (resulting string=w497:string)  [unwired: 2 in, 1 out]
                        n195 = Increment(x=w500) -> (x+1=w501:i32)
                        n196 = Not Equal?(x=w492, y=w496) -> (x != y?=w495:bool)
                        n197 = Concatenate Strings(w497, "\r") -> (w487:string)
                        n198 = local read "Remote Mode"() -> (w486:u16)
                        n199 = Select(t=w501, s=w495, f=0) -> (s? t:f=w494:i32)
                        n200 = call "SSI_Control.vi"("Write Buffer"=w487, "Remote Mode"=w486, "Error in (no error)"=w489, "Control"=w483, "Connection ID in"=w484, "VISA resource name"=w482) -> ("Error out"=w488:errorcluster, "Connection ID out"=w480:refnum<k5>, "VISA resource  out"=w481:refnum<visa-resource-name>)  [unwired: 2 in, 1 out]
                      }
                    }
                  }
                  frame #2 {
                    n201 = local read "Sweep"() -> (w512:u16)
                    n202 = Equal To 0?(x=w512) -> (x = 0?=w511:bool)
                    n203 = Select(t=w513, s=w514, f=u16 0) -> (s? t:f=w516:i32)
                    n204 = Select(t=T1."Trig In Type" ("function"), s=w511, f=T1."Int_Sweep_Trig In" ("function")) -> (s? t:f=w510:T1)
                  }
                }
                n205 = local read "Step Time(ms)"() -> (w406:i32)
                n206 = Wait (ms)(milliseconds to wait=w406) -> ()  [unwired: 1 out]
              }
            }
          }
          event "Stop Frequency(Hz)", "Linear Step Frequency(Hz)", "Log Step Percent(%)", "Sweep Run Mode", "Sweep Mode", "Start Frequency(Hz)": Value Change {
            (unwired) dbl[] [] ("历史数据")
            n207 = event-data() -> ()  [unwired: 1 in, 5 out]
            n208 = Wait (ms)(milliseconds to wait=u32 10 ("等待时间（毫秒）")) -> ()  [unwired: 1 out]
          }
          event "Parameter Index": Value Change {
            (unwired) dbl[] [] ("历史数据")
            n209 = event-data() -> ()  [unwired: 1 in, 5 out]
            n210 = Wait (ms)(milliseconds to wait=u32 10 ("等待时间（毫秒）")) -> ()  [unwired: 1 out]
          }
          event "Trig Mode": Value Change {
            (unwired) dbl[] [] ("历史数据")
            n211 = event-data() -> ()  [unwired: 1 in, 5 out]
            n212 = local read "Trig Mode"() -> (w552:u8)
            n213 = local read "Remote Mode"() -> (w553:u16)
            n214 = call "OE2031&OE2041_Configure Trig.vi"("Trig Mode"=w552, "Error in (no error)"=w556, "Remote Mode"=w553, "Connection ID in"=w555, "VISA resource name"=w554) -> ("Error out"=w551:errorcluster, "Connection ID out"=w550:refnum<k5>, "VISA resource  out"=w549:refnum<visa-resource-name>)  [unwired: 3 in, 1 out]
            n215 = local read "Trig Mode"() -> (w544:u8)
            n216 = local read "Sweep"() -> (w540:u16)
            n217 = Less Or Equal?(x=w544, y=u8 2) -> (x <= y?=w543:bool)
            n218 = Select(t=T2."Enabled" ("禁用"), s=w543, f=T2."Disabled and Grayed Out") -> (s? t:f=w547:T2)
            n219 = Not Equal To 0?(x=w540) -> (x != 0?=w539:bool)
            n220 = property on="Sweep" class="Ring (严格)"("DisabledEnum"=w547) -> ()  [unwired: 2 in, 2 out]
            n221 = And(x=w543, y=w539) -> (x .and. y?=w542:bool)
            n222 = Wait (ms)(milliseconds to wait=u32 10 ("等待时间（毫秒）")) -> ()  [unwired: 1 out]
            n223 = property on="选项卡控件" class="TabCtl (严格)"("Visible"=w542) -> ()  [unwired: 2 in, 2 out]
            n224 = property on="Interval Count" class="DigNum (严格)"("Visible"=w542) -> ()  [unwired: 2 in, 2 out]
            n225 = case shown="真" w542 {
              frame False {
              }
              frame True {
                n226 = local read "Trig Mode"() -> (w561:u8)
                n227 = local read "Sweep Mode"() -> (w566:u16)
                n228 = Equal To 0?(x=w561) -> (x = 0?=w562:bool)
                n229 = Equal To 0?(x=w566) -> (x = 0?=w567:bool)
                n230 = case shown="真" w562 {
                  tunnel: [T2."Disabled and Grayed Out" ("禁用") T2."Enabled" ("禁用")] -> w564
                  tunnel: [T2."Enabled" ("禁用") T2."Disabled and Grayed Out" ("禁用")] -> w563
                  frame False {
                  }
                  frame True {
                  }
                }
                n231 = Not(x=w567) -> (.not. x?=w565:bool)
                n232 = property on="Linear Step Frequency(Hz)" class="DigNum (严格)"("Visible"=w567) -> ()  [unwired: 2 in, 2 out]
                n233 = property on="Log Step Percent(%)" class="DigNum (严格)"("Visible"=w565) -> ()  [unwired: 2 in, 2 out]
                n234 = property on="Step Time(ms)" class="DigNum (严格)"("DisabledEnum"=w564) -> ()  [unwired: 2 in, 2 out]
                n235 = property on="Interval Count" class="DigNum (严格)"("DisabledEnum"=w563) -> ()  [unwired: 2 in, 2 out]
              }
            }
          }
          event "Ref_Source": Value Change {
            (unwired) dbl[] [] ("历史数据")
            w589 = u16 0 items=["Write", "Read"] ("Control")
            n236 = event-data() -> ()  [unwired: 1 in, 5 out]
            n237 = local read "Remote Mode"() -> (w575:u16)
            n238 = local read "Ref_Source"() -> (w587:u8)
            n239 = Format Into String(format string="FMOD %d;" ("格式字符串"), w587) -> (resulting string=w586:string)  [unwired: 2 in, 1 out]
            n240 = Concatenate Strings(w586, "\r") -> (w590:string)
            n241 = call "SSI_Control.vi"("Write Buffer"=w590, "Remote Mode"=w575, "Error in (no error)"=w581, "Control"=w589, "Connection ID in"=w579, "VISA resource name"=w578) -> ("Error out"=w580:errorcluster, "Connection ID out"=w576:refnum<k5>, "VISA resource  out"=w577:refnum<visa-resource-name>)  [unwired: 2 in, 1 out]
            n242 = Wait (ms)(milliseconds to wait=u32 10 ("等待时间（毫秒）")) -> ()  [unwired: 1 out]
          }
          event "Sweep": Value Change {
            (unwired) dbl[] [] ("历史数据")
            n243 = event-data() -> ()  [unwired: 1 in, 5 out]
            n244 = local read "Sweep"() -> (w600:u16)
            n245 = Not Equal To 0?(x=w600) -> (x != 0?=w591:bool)
            n246 = case shown="真" w591 {
              frame False {
              }
              frame True {
                n247 = local read "Trig Mode"() -> (w601:u8)
                n248 = local read "Sweep Mode"() -> (w606:u16)
                n249 = Equal To 0?(x=w601) -> (x = 0?=w602:bool)
                n250 = Equal To 0?(x=w606) -> (x = 0?=w607:bool)
                n251 = case shown="真" w602 {
                  tunnel: [T2."Disabled and Grayed Out" ("禁用") T2."Enabled" ("禁用")] -> w604
                  tunnel: [T2."Enabled" ("禁用") T2."Disabled and Grayed Out" ("禁用")] -> w603
                  frame False {
                  }
                  frame True {
                  }
                }
                n252 = Not(x=w607) -> (.not. x?=w605:bool)
                n253 = property on="Linear Step Frequency(Hz)" class="DigNum (严格)"("Visible"=w607) -> ()  [unwired: 2 in, 2 out]
                n254 = property on="Log Step Percent(%)" class="DigNum (严格)"("Visible"=w605) -> ()  [unwired: 2 in, 2 out]
                n255 = property on="Step Time(ms)" class="DigNum (严格)"("DisabledEnum"=w604) -> ()  [unwired: 2 in, 2 out]
                n256 = property on="Interval Count" class="DigNum (严格)"("DisabledEnum"=w603) -> ()  [unwired: 2 in, 2 out]
              }
            }
            n257 = property on="选项卡控件" class="TabCtl (严格)"("Visible"=w591) -> ()  [unwired: 2 in, 2 out]
            n258 = property on="Interval Count" class="DigNum (严格)"("Visible"=w591) -> ()  [unwired: 2 in, 2 out]
          }
        }
        n259 = local read "Connect"() -> (w31:bool)
        n260 = Not(x=w31) -> (.not. x?=w42:bool)
        n261 = Or(x=w28, y=w42) -> (x .or. y?=w41:bool)
      }
      n262 = call "SSI_Close.vi"("Error in (no error)"=w21, "Connection ID in"=w17, "VISA resource name"=w16) -> ("Error out"=→"Error out":errorcluster)  [unwired: 4 in]
    }
  }
